vi "AprilTag ID List (Tag25h9).vi"() -> (0 "Tag IDs":i32[](array[numeric]))   [LabVIEW 2020, in "feature_detection.lvlib"]
doc: "Get a list of the IDs for a AprilTag Tag Family. This can be used with Generate AprilTag Image Data.vi to generate some or all of the Tags in that family."
uses:
  feature_detection.lvlib
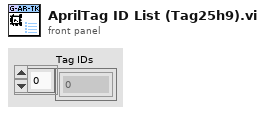
[diagram p1: front panel]
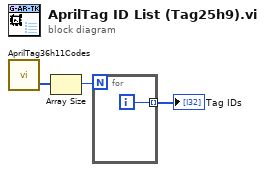
[diagram p0: block diagram]
diagram:
  n1 = call "AprilTag36h11Codes.vi"() -> ("Codes"=w2:i64[])  [unwired: 2 in, 1 out]
  n2 = Array Size(array=w2) -> (size(s)=w3:i32)
  n3 = for {
    N: w3 -> [_]
    tunnel: [w4] -> w1 mode=indexing
    i -> [w4]
  }
  "Tag IDs" <- w1
